vi "PI-C867-JoystickState.vi"(8 "error in":errorcluster, 10 "JoystickID to query":i32[](array[numeric])=[3], 11 "System no.":i32=2 min=1 max=4 step=1) -> (0 "error out":errorcluster, 3 "State":bool[][](array[boolean]))   [LabVIEW 2014]
doc: "This Vi checks the 6 button state of the Joystick"
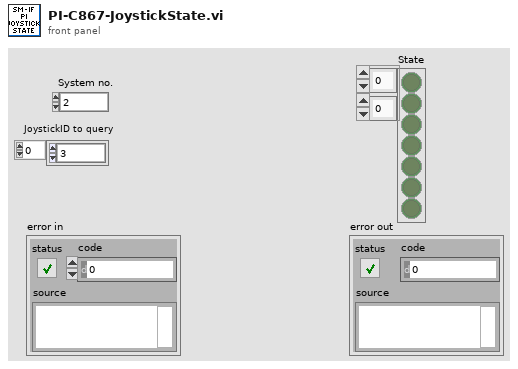
[diagram p1: front panel]
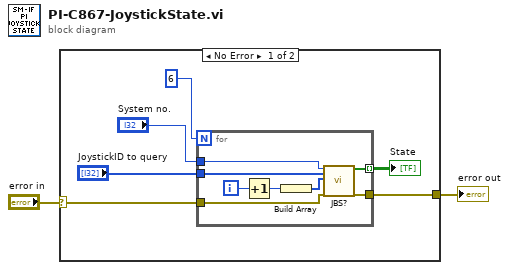
[diagram p0: block diagram]
diagram:
  n1 = case shown="No Error" "error in" {
    selector: "error in" -> [w3 w17]
    tunnel: [w5 w17] -> w2
    frame No Error {
      n2 = for {
        N: 6 -> [_]
        tunnel: w3 -> [w16]
        tunnel: "System no." -> [w15]
        tunnel: "JoystickID to query" -> [w14]
        tunnel: [w11] -> w4 mode=indexing
        tunnel: [w10] -> w5
        i -> [w13]
        n3 = Increment(x=w13) -> (x+1=w9:i32)
        n4 = Build Array(w9) -> (w12:i32[])
        n5 = call "JBS?.vi"("System no."=w15, "JoystickID to query"=w14, "Joystick button"=w12, "error in"=w16) -> ("State"=w11:bool[], "error out"=w10:errorcluster)  [unwired: 14 in]
      }
      "State" <- w4
    }
    frame Error {
    }
  }
  "error out" <- w2
